vi "Configure Calc dB dBm.vi"(8 "error in (no error)":errorcluster, 9 "DB D Constant (1)":dbl=1.0 min=1e-14 max=999999000000.0 step=1e-14 format="%_6g", 10 "Calculate DB  (0: Off)":u16(ring) items=["Off", "dB On", "dBm On"], 11 "VISA resource name":refnum<visa-resource-name>) -> (0 "error out":errorcluster, 3 "VISA resource name out":refnum<visa-resource-name>)   [LabVIEW 2017, in "ADCMT7451_ADC.lvlib"]
doc: "Enables or disables dB/dBm calculation."
uses:
  ADCMT7451_ADC.lvlib
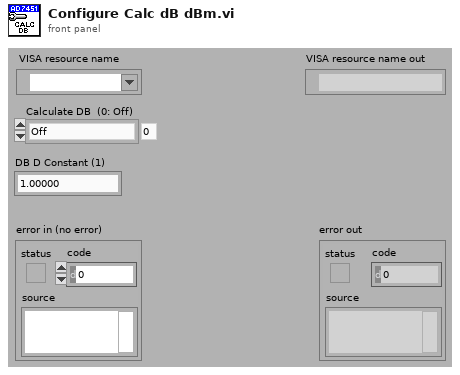
[diagram p1: front panel]
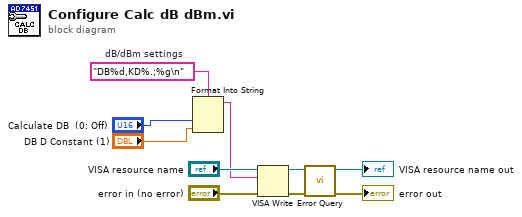
[diagram p0: block diagram]
diagram:
  w4 = "DB%d,KD%.;%g\n"  # dB/dBm settings
  n1 = Format Into String(format string=w4, "Calculate DB  (0: Off)", "DB D Constant (1)") -> (resulting string=w1:string)  [unwired: 2 in, 1 out]
  n2 = VISA Write(VISA resource name="VISA resource name", write buffer=w1, error in (no error)="error in (no error)") -> (VISA resource name out=w6:refnum<visa-resource-name>, error out=w5:errorcluster)  [unwired: 1 out]
  n3 = call "Error Query.vi"("error in (no error)"=w5, "VISA resource name"=w6) -> ("error out"=→"error out":errorcluster, "VISA resource name out"=→"VISA resource name out":refnum<visa-resource-name>)  [unwired: 6 in, 2 out]
